vi "WriteAItoSV.vi"(8 "error in (no error)":errorcluster, 9 "Timeout in ms (100)":i32=100, 10 "AI Data":T1[](array[typedef]), 11 "SharedVariableRefnums":refnum<k21>[](array[refnum])) -> (0 "error out":errorcluster)   [LabVIEW 2013]
uses:
  AI_Data.ctl
  <vilib>/Utility/error.llb/Error Cluster From Error Code.vi
  <vilib>/ErrorRing/Error Ring.xnode
  <resource>/objmgr/ni.var.rc
  <vilib>/Utility/Variable/NI_VariableUtilities.lvlib
  NI Card.lvclass
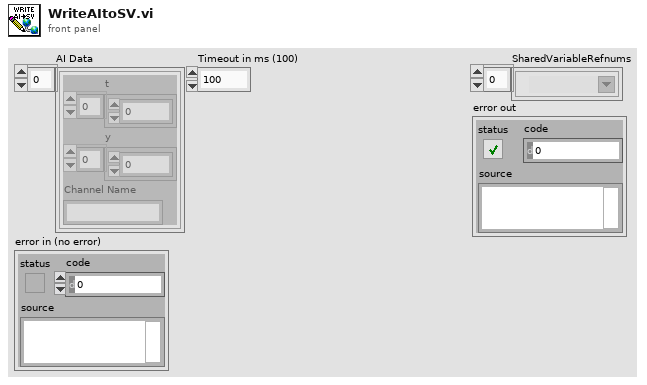
[diagram p1: front panel]
types:
  T1 = typedef "NI Card.lvclass/AI_Data.ctl" = cluster{"t":dbl[], "y":dbl[], "Channel Name":string}
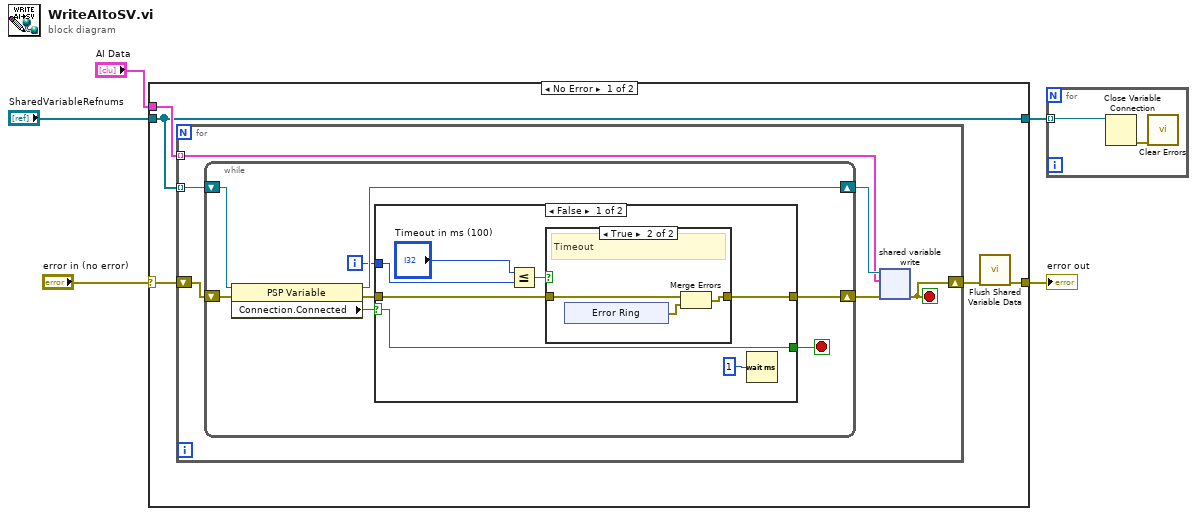
[diagram p0: block diagram]
diagram:
  n1 = case shown="No Error" "error in (no error)" {
    selector: "error in (no error)" -> [w9 w43]
    tunnel: [w6 w43] -> w1
    tunnel: "SharedVariableRefnums" -> [w8 w42]
    tunnel: "AI Data" -> [w10 _]
    tunnel: [w8 w42] -> w2
    frame No Error {
      n2 = for {
        tunnel: w8 -> [w16] mode=indexing
        tunnel: w10 -> [w11] mode=indexing
        shift-right: [w12] -> w7
        shift-left: w9 -> [w15]
        stop <- w12 stop-if-true
        n3 = while {
          shift-right: [w23] -> w14
          shift-left: w16 -> [w24]
          shift-right: [w20] -> w13
          shift-left: w15 -> [w22]
          i -> [w17]
          stop <- w18 stop-if-true
          n4 = property class="PSP Variable"(reference=w24, error in=w22) -> (reference out=w23:refnum<k21>, error out=w21:errorcluster, "Connection.Connected"=w19:bool)
          n5 = case shown="False" w19 {
            selector: w19 -> [w30 w40]
            tunnel: w21 -> [w26 w41]
            tunnel: [w25 w41] -> w20
            tunnel: [w30 w40] -> w18
            tunnel: w17 -> [w28 _]
            frame False {
              n6 = Less Or Equal?(x="Timeout in ms (100)", y=w28) -> (x <= y?=w27:bool)
              n7 = case shown="True" w27 {
                tunnel: w26 -> [w32 w35]
                tunnel: [w32 w34] -> w25
                frame False {
                }
                frame True {
                  # "Timeout"
                  n8 = xnode "Error Ring"() -> ("error out"=w33:errorcluster)
                  n9 = Merge Errors(w35, w33) -> (w34:errorcluster)
                }
              }
              n10 = Wait (ms)(milliseconds to wait=u32 1) -> ()  [unwired: 1 out]
            }
            frame True {
            }
          }
        }
        n11 = shared-variable-write(w14, w13, w11) -> (w12:errorcluster)  [unwired: 1 out]
      }
      n12 = call <vilib>:"Flush Shared Variable Data.vi"("error in (no error)"=w7) -> ("error out"=w6:errorcluster)  [unwired: 10 in]
    }
    frame Error {
    }
  }
  "error out" <- w1
  n13 = for {
    tunnel: w2 -> [w44] mode=indexing
    n14 = Close Variable Connection(11:w44) -> (0:w45:errorcluster)  [unwired: 1 in]
    n15 = call <vilib>:"Clear Errors.vi"("error in (no error)"=w45) -> ()  [unwired: 6 in, 1 out]
  }
